vi "Example Tractor Lights 2.vi"() -> ()   [LabVIEW 2014]
uses:
  LabVIEW-Universal-Transcriptor-ServoLibrary/ServoDatatype.lvclass
panel:
  in  "Error In":errorcluster
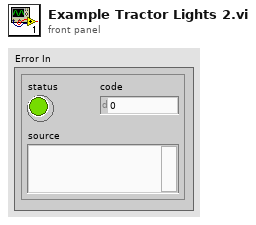
[diagram p1: front panel]
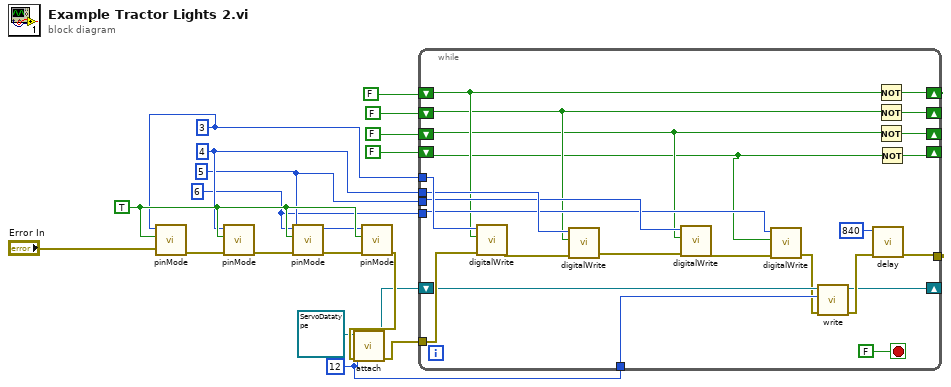
[diagram p0: block diagram]
diagram:
  w2 = 12 ("pin number")
  w9 = 3 ("pin number")
  w8 = 4 ("pin number")
  w7 = 5 ("pin number")
  w6 = 6 ("pin number")
  w15 = TRUE ("output?")
  n1 = call <vilib>:"pinMode.vi"("Error In"="Error In", "output?"=w15, "pin number"=w9) -> ("Error Out"=w18:errorcluster)  [unwired: 8 in]
  n2 = call <vilib>:"pinMode.vi"("Error In"=w18, "output?"=w15, "pin number"=w8) -> ("Error Out"=w17:errorcluster)  [unwired: 8 in]
  n3 = call <vilib>:"pinMode.vi"("Error In"=w17, "output?"=w15, "pin number"=w7) -> ("Error Out"=w16:errorcluster)  [unwired: 8 in]
  n4 = call <vilib>:"pinMode.vi"("Error In"=w16, "output?"=w15, "pin number"=w6) -> ("Error Out"=w5:errorcluster)  [unwired: 8 in]
  n5 = call-dynamic "attach.vi"("error in (no error)"=w5, "pin number"=w2, "Servo in"=refnum<class "ServoDatatype.lvclass"> refnum) -> ("error out"=w4:errorcluster, "Servo out"=w1:refnum<class "ServoDatatype.lvclass">)  [unwired: 6 in, 1 out]
  n6 = while {
    shift-right: [w42] -> _
    shift-left: FALSE ("output?") -> [w31]
    shift-right: [w41] -> _
    shift-left: FALSE ("output?") -> [w30]
    shift-right: [w40] -> _
    shift-left: FALSE ("output?") -> [w29]
    shift-right: [w39] -> _
    shift-left: FALSE ("output?") -> [w28]
    tunnel: w9 -> [w35]
    tunnel: w8 -> [w34]
    tunnel: w7 -> [w33]
    tunnel: w6 -> [w32]
    tunnel: [w26] -> _
    tunnel: w4 -> [w24]
    tunnel: w2 -> [w23]
    shift-right: [w19] -> _
    shift-left: w1 -> [w22]
    stop <- FALSE stop-if-true
    n7 = call <vilib>:"digitalWrite.vi"("Error In"=w24, "value"=w31, "pin number"=w35) -> ("Error Out"=w36:errorcluster)  [unwired: 8 in]
    n8 = call <vilib>:"digitalWrite.vi"("Error In"=w36, "value"=w30, "pin number"=w34) -> ("Error Out"=w37:errorcluster)  [unwired: 8 in]
    n9 = call <vilib>:"digitalWrite.vi"("Error In"=w37, "value"=w29, "pin number"=w33) -> ("Error Out"=w38:errorcluster)  [unwired: 8 in]
    n10 = call <vilib>:"digitalWrite.vi"("Error In"=w38, "value"=w28, "pin number"=w32) -> ("Error Out"=w21:errorcluster)  [unwired: 8 in]
    n11 = call-dynamic "write.vi"("error in (no error)"=w21, "value"=w23, "ServoDatatype in"=w22) -> ("error out"=w20:errorcluster, "ServoDatatype out"=w19:refnum<class "ServoDatatype.lvclass">)  [unwired: 7 in]
    n12 = call <vilib>:"delay.vi"("Error In"=w20, "time (ms)"=840) -> ("Error Out"=w26:errorcluster)  [unwired: 9 in]
    n13 = Not(x=w31) -> (.not. x?=w42:bool)
    n14 = Not(x=w30) -> (.not. x?=w41:bool)
    n15 = Not(x=w29) -> (.not. x?=w40:bool)
    n16 = Not(x=w28) -> (.not. x?=w39:bool)
  }
